vi "TransformMap.vi"() -> ()   [LabVIEW 2009]
uses:
  <vilib>/vision/NI_Vision_Development_Module.lvlib
panel:
  in  "Calibration Learn Setup":T1={"Distortion"=0, "Corrected Image Scaling"=0, "Corrected Image Learn ROI"=2, "Learn Error Map?"=FALSE, "Learn Correction Table?"=FALSE} {"Corrected Image Learn ROI" items=["Full Image ", "Calibration ROI", "ROI", "Calibration AND ROI", "Calibration OR ROI"]; "Corrected Image Scaling" items=["Scale to Preserve Area", "Scale to Fit"]; "Distortion" items=["Perspective", "Nonlinear"]}
  in  "Grid Descriptor 2":T2={"X Step"=0.0, "Y Step"=0.0, "Unit"=enum."Undefined", "Threshold Range"={"Lower value"=0.0, "Upper value"=128.0}} {"Threshold Range"."Upper value" format="%.2f"; "Threshold Range"."Lower value" format="%.2f"; "Y Step" format="%.2f"; "X Step" format="%.2f"}
  out "'input Image 2":T4(plugin-control)
  in  "Input Image Path":path=path "C:/Documents and Settings/dgrieneisen/My Documents/Robotics/Athena/image2004.jpg"
  out "'input Image":T4(plugin-control)
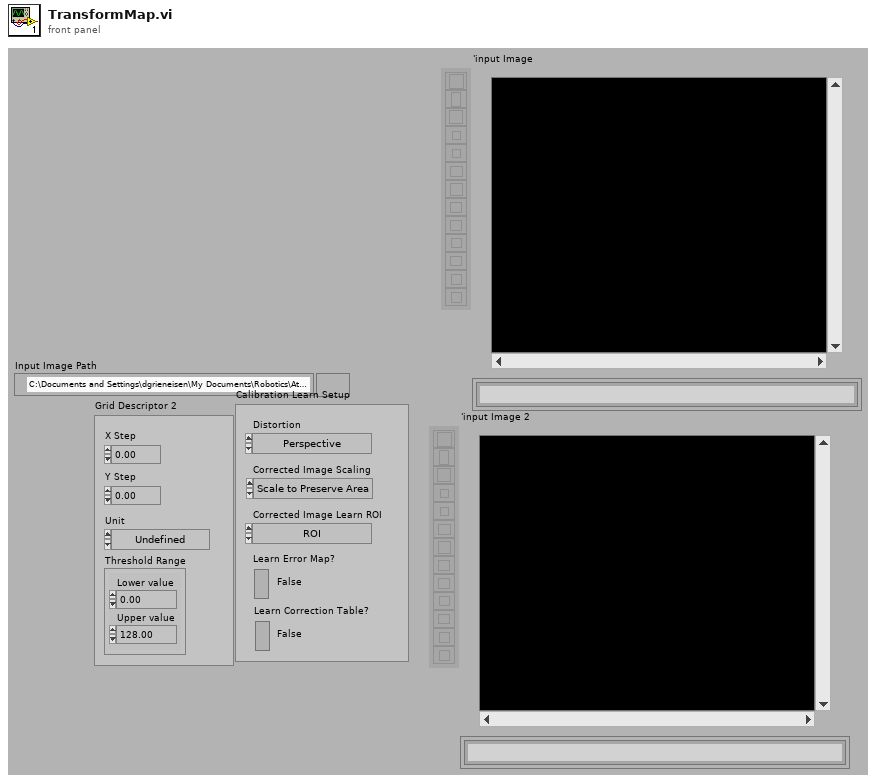
[diagram p1: front panel]
types:
  T1 = cluster{"Distortion":u32, "Corrected Image Scaling":u32, "Corrected Image Learn ROI":u32, "Learn Error Map?":bool, "Learn Correction Table?":bool}
  T2 = typedef "Grid Descriptor" = cluster{"X Step":sgl, "Y Step":sgl, "Unit":T3, "Threshold Range":cluster{"Lower value":sgl, "Upper value":sgl}}
  T3 = typedef "Image Unit" = enum32{"Undefined", "Angström", "Micrometer", "Millimeter", "Centimeter", "Meter", "Kilometer", "Microinch", "Inch", "Feet", "Nautical miles", "Standard miles", "Steps"}
  T4 = typedef "IMAQ Image.ctl" = refnum<image>
  T5 = cluster{"Origin Pixel":cluster{"X":sgl, "Y":sgl}, "Angle Relative to Horizontal (deg)":sgl, "Axis Reference":u32}
  T6 = typedef "Image Type" = u32
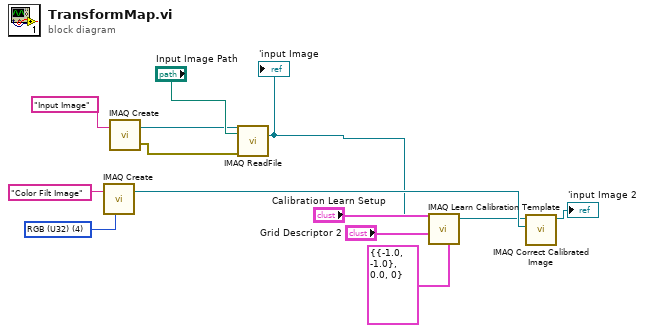
[diagram p0: block diagram]
diagram:
  w12 = T6 4 items=["Grayscale (U8)", "Grayscale (I16)", "Grayscale (SGL)", "Complex (CSG)", "RGB (U32)", "HSL (U32)", "RGB (U64)", "Grayscale (U16)"] ("Image Type")
  n1 = call "IMAQ Create"("Image Name"="Color Filt Image", "Image Type"=w12) -> ("New Image"=w4:T4)  [unwired: 2 in, 2 out]
  n2 = call "IMAQ Create"("Image Name"="Input Image") -> ("New Image"=w8:T4, "error out"=w9:errorcluster)  [unwired: 3 in, 1 out]
  n3 = call "IMAQ ReadFile"("File Path"="Input Image Path", "error in (no error)"=w9, "Image"=w8) -> ("Image Out"=w2:T4)  [unwired: 4 in, 4 out]
  "'input Image" <- w2
  n4 = call "IMAQ Learn Calibration Template"("Calibration Axis Info"=T5 {"Origin Pixel"={"X"=-1.0, "Y"=-1.0}, "Angle Relative to Horizontal (deg)"=0.0, "Axis Reference"=0}, "Grid Descriptor"="Grid Descriptor 2", "Calibration Learn Setup"="Calibration Learn Setup", "Image"=w2) -> ("Calibrated Image"=w3:T4)  [unwired: 5 in, 2 out]
  n5 = call "IMAQ Correct Calibrated Image"("Image Dst"=w4, "Image Src"=w3) -> ("Corrected Image"=→"'input Image 2":T4)  [unwired: 8 in, 1 out]
